vi "4-4.vi"() -> ()   [LabVIEW 2017]
panel:
  in  "最低温度":dbl
  in  "最高温度":dbl
  in  "温度":dbl
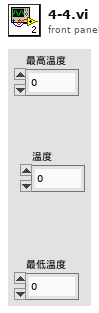
[diagram p1: front panel]
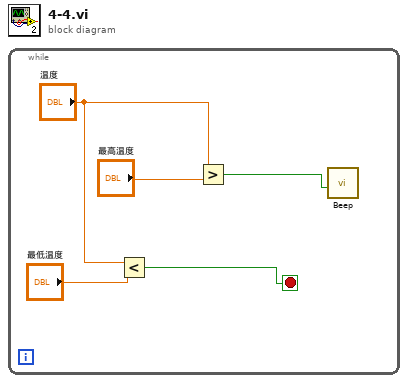
[diagram p0: block diagram]
diagram:
  n1 = while {
    stop <- w1 stop-if-true
    n2 = Less?(x="温度", y="最低温度") -> (x < y?=w1:bool)
    n3 = Greater?(x="温度", y="最高温度") -> (0:w2:bool)
    n4 = call <vilib>:"Beep.vi"("use system alert? (T)"=w2) -> ()  [unwired: 11 in]
  }
